vi "ROI_Analysis.vi"(8 "error in (no error)":errorcluster, 10 "ROI":T1 {"Contours"."Type" items=["No Selection", "Point", "Line", "Rectangle", "Oval", "Polygon", "Freehand Region", "Annulus", "Unused2", "Unused3", "Broken Line", "Freehand Line", "Rotated Rectangle"]}, 11 "Image In":T2) -> (0 "error out":errorcluster, 2 "ROI Results":dbl, 3 "ROI Snippet Out":T2)   [LabVIEW 2012]
uses:
  <vilib>/vision/Image Controls.llb/IMAQ Image.ctl
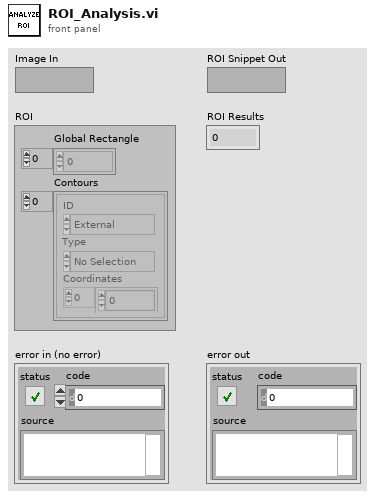
[diagram p1: front panel]
types:
  T1 = typedef "ROI Descriptor" = cluster{"Global Rectangle":i32[], "Contours":cluster{"ID":enum32{"External", "Internal"}, "Type":u32, "Coordinates":i32[]}[]}
  T2 = typedef "IMAQ Image.ctl" = refnum<image>
  T3 = typedef "Image Type" = u32
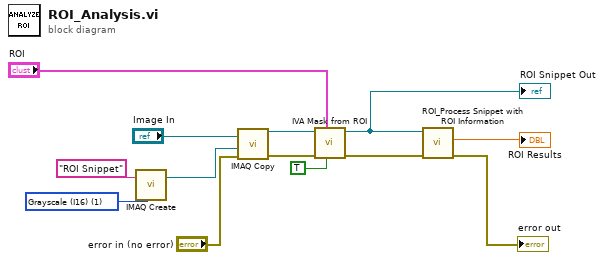
[diagram p0: block diagram]
diagram:
  w12 = T3 1 items=["Grayscale (U8)", "Grayscale (I16)", "Grayscale (SGL)", "Complex (CSG)", "RGB (U32)", "HSL (U32)", "RGB (U64)", "Grayscale (U16)"] ("Image Type")
  n1 = call "IMAQ Create"("Image Name"="ROI Snippet", "Image Type"=w12) -> ("New Image"=w13:T2)  [unwired: 2 in, 2 out]
  n2 = call "IMAQ Copy"("error in (no error)"="error in (no error)", "Image Dst"=w13, "Image Src"="Image In") -> ("error out"=w6:errorcluster, "Image Dst Out"=w7:T2)  [unwired: 3 in]
  n3 = call <vilib>:"IVA Mask from ROI.vi"("Shrink"=TRUE, "ROI Descriptor"="ROI", "error in (no error)"=w6, "Image Src"=w7) -> ("error out"=w1:errorcluster, "Image Out"=w10:T2)  [unwired: 1 in, 5 out]
  "ROI Snippet Out" <- w10
  n4 = call "ROI_Process Snippet with ROI Information.vi"("error in (no error)"=w1, "ROI Snippet"=w10) -> ("error out"=→"error out":errorcluster, "ROI Information"=→"ROI Results":dbl)  [unwired: 8 in]
